vi "test_ini — 3.vi"() -> ()   [LabVIEW 2016]
uses:
  <vilib>/Utility/config.llb/Write Key (Double).vi
  <vilib>/Utility/config.llb/Write Key (Boolean).vi
  <vilib>/Utility/config.llb/Read Key (Double).vi
  <vilib>/Utility/config.llb/Read Key (Boolean).vi
  <vilib>/Utility/config.llb/NI_LVConfig.lvlib
panel:
  in  "stop":bool
  in  "write":bool
  in  "Slide":dbl(slide) scale=0.0..10.0
  in  "GAS":bool
  in  "I":dbl
  in  "U":dbl
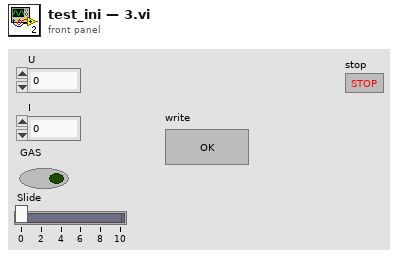
[diagram p1: front panel]
types:
  T1 = enum16{"open", "replace", "create", "open or create", "replace or create", "replace or create with confirmation"}
  T2 = typedef "NI_LVConfig.lvlib/Config Data RefNum.ctl" = refnum<k1>
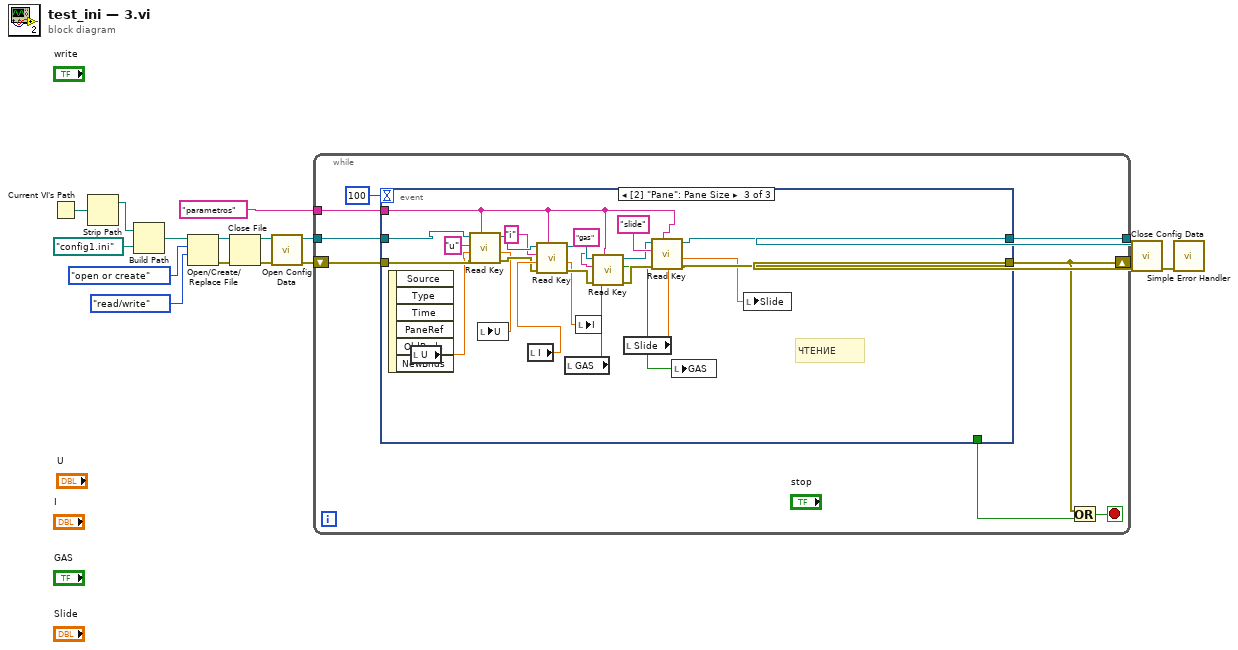
[diagram p0: block diagram]
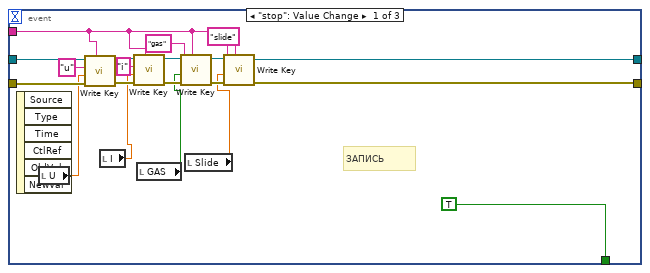
[diagram p2: hidden frame]
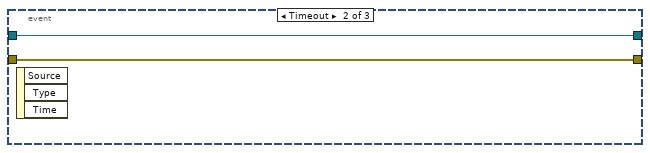
[diagram p3: hidden frame]
diagram:
  n1 = Current VI's Path() -> (path=w16:path)
  n2 = Strip Path(path=w16) -> (stripped path=w15:path)  [unwired: 1 out]
  n3 = Build Path(base path=w15, name or relative path=path "config1.ini") -> (appended path=w13:path)
  n4 = Open/Create/Replace File(file path (use dialog)=w13, operation (0:open)=T1."open or create", access (0:read/write)=enum16{"read/write", "read-only", "write-only"}."read/write") -> (refnum out=w10:refnum<file>, error out=w9:errorcluster)  [unwired: 3 in, 1 out]
  n5 = Close File(refnum=w10, error in=w9) -> (path=w8:path, error out=w1:errorcluster)
  n6 = call <vilib>:"Open Config Data.vi"("error in (no error)"=w1, "configuration file path"=w8) -> ("error out"=w6:errorcluster, "refnum"=w7:T2)  [unwired: 7 in, 1 out]
  n7 = while {
    shift-right: [w20] -> w5
    shift-left: w6 -> [w21]
    tunnel: w7 -> [w22]
    tunnel: [w19] -> w3
    tunnel: "parametros" ("section") -> [w18]
    stop <- w24 stop-if-true
    n8 = event shown="[2] \"Pane\": Pane Size" {
      selector: _ -> [_ _ _]
      dyn-events: _ -> [_ _ _]
      timeout: 100 -> [_ _ _]
      tunnel: w22 -> [w44 w46 w67]
      tunnel: w21 -> [w43 w45 w68]
      tunnel: [w37 w45 w64] -> w20
      tunnel: [w38 w46 w65] -> w19
      tunnel: w18 -> [w26 _ w58]
      tunnel: [TRUE _ _] -> w17
      event "stop": Value Change {
        # "ЗАПИСЬ"
        n9 = event-data() -> ()  [unwired: 1 in, 6 out]
        n10 = local read "U"() -> (w41:dbl)
        n11 = call-poly <vilib>:"Write Key.vi"("section"=w26, "error in (no error)"=w43, "value"=w41, "key"="u", "refnum"=w44) -> ("error out"=w39:errorcluster, "refnum out"=w40:T2)  [unwired: 4 in, 1 out]
        n12 = local read "I"() -> (w29:dbl)
        n13 = call-poly <vilib>:"Write Key.vi"("section"=w26, "error in (no error)"=w39, "value"=w29, "key"="i", "refnum"=w40) -> ("error out"=w33:errorcluster, "refnum out"=w34:T2)  [unwired: 4 in, 1 out]
        n14 = local read "GAS"() -> (w28:bool)
        n15 = call-poly <vilib>:"Write Key.vi"("section"=w26, "error in (no error)"=w33, "value"=w28, "key"="gas", "refnum"=w34) -> ("error out"=w36:errorcluster, "refnum out"=w35:T2)  [unwired: 4 in, 1 out]
        n16 = local read "Slide"() -> (w27:dbl)
        n17 = call-poly <vilib>:"Write Key.vi"("section"=w26, "error in (no error)"=w36, "value"=w27, "key"="slide", "refnum"=w35) -> ("error out"=w37:errorcluster, "refnum out"=w38:T2)  [unwired: 4 in, 1 out]
      }
      event Timeout {
        n18 = event-data() -> ()  [unwired: 1 in, 3 out]
      }
      event Pane Size {
        # "ЧТЕНИЕ"
        n19 = event-data() -> ()  [unwired: 1 in, 6 out]
        n20 = local read "U"() -> (w66:dbl)
        n21 = call-poly <vilib>:"Read Key.vi"("section"=w58, "error in (no error)"=w68, "default value"=w66, "key"="u", "refnum"=w67) -> ("error out"=w60:errorcluster, "value"=w50:dbl, "refnum out"=w61:T2)  [unwired: 3 in, 1 out]
        n22 = local write "U"(w50) -> ()
        n23 = local read "I"() -> (w62:dbl)
        n24 = call-poly <vilib>:"Read Key.vi"("section"=w58, "error in (no error)"=w60, "default value"=w62, "key"="i", "refnum"=w61) -> ("error out"=w54:errorcluster, "value"=w49:dbl, "refnum out"=w55:T2)  [unwired: 3 in, 1 out]
        n25 = local read "GAS"() -> (w52:bool)
        n26 = local write "I"(w49) -> ()
        n27 = call-poly <vilib>:"Read Key.vi"("section"=w58, "error in (no error)"=w54, "default value"=w52, "key"="gas", "refnum"=w55) -> ("error out"=w57:errorcluster, "found?"=w48:bool, "refnum out"=w56:T2)  [unwired: 3 in, 1 out]
        n28 = local read "Slide"() -> (w51:dbl)
        n29 = call-poly <vilib>:"Read Key.vi"("section"=w58, "error in (no error)"=w57, "default value"=w51, "key"="slide", "refnum"=w56) -> ("error out"=w64:errorcluster, "value"=w47:dbl, "refnum out"=w65:T2)  [unwired: 3 in, 1 out]
        n30 = local write "GAS"(w48) -> ()
        n31 = local write "Slide"(w47) -> ()
      }
    }
    n32 = Or(x=w20, y=w17) -> (x .or. y?=w24:bool)
  }
  n33 = call <vilib>:"Close Config Data.vi"("error in (no error)"=w5, "refnum"=w3) -> ("error out"=w4:errorcluster)  [unwired: 8 in, 1 out]
  n34 = call <vilib>:"Simple Error Handler.vi"("error in (no error)"=w4) -> ()  [unwired: 4 in, 5 out]
